vi "Synchronize Control Panel.vi"(8 "error in (no error)":errorcluster, 11 "Device in":refnum<class "Cryo-Con-22C.lvclass">) -> (0 "error out":errorcluster, 3 "Device out":refnum<class "Cryo-Con-22C.lvclass">)   [LabVIEW 2015, in "Cryo-Con-22C.lvclass"]
uses:
  Cryo-Con-22C.lvclass
  Cryo-Con Front Panel Data.ctl
  Cryo-con Heater Ranges.ctl
  Cry-Con Loop Type.ctl
  Instrument/Read VISA Resource.vi
  Instrument/Write VISA Resource.vi
  OO Devices/Device/Device.lvclass
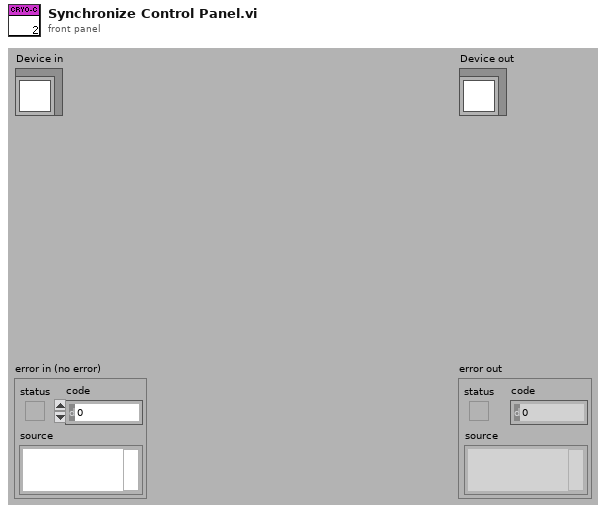
[diagram p1: front panel]
types:
  T1 = typedef "Cryo-Con Front Panel Data.ctl" = cluster{"Channels to measure":string[], "Record heater":bool, "Set point":dbl, "Heater Range":T2, "Control":bool, "Loop type":T3, "Ramp rate,\n K/min":dbl, "Control Channel":string, "P":dbl, "I":dbl, "D":dbl, "Manual %":u16}
  T2 = typedef "Cryo-con Heater Ranges.ctl" = enum16{"25W", "2.5W", "0.25W"}
  T3 = typedef "Cry-Con Loop Type.ctl" = enum16{"Off", "PID", "Manual", "PID Table", "PID Ramp", "PID Table Ramp"}
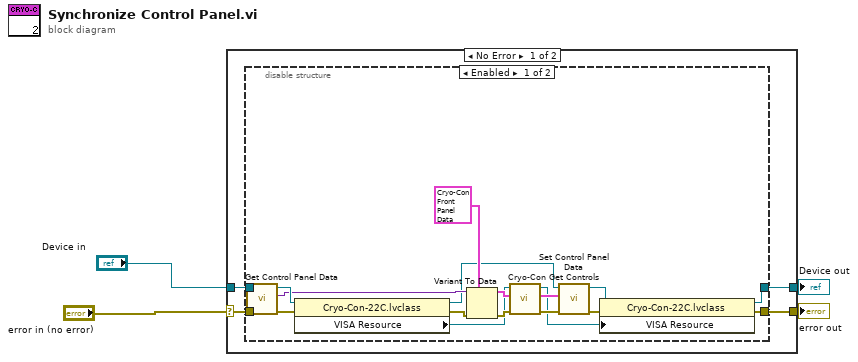
[diagram p0: block diagram]
diagram:
  n1 = case shown="No Error" "error in (no error)" {
    selector: "error in (no error)" -> [w7 w30]
    tunnel: [w6 w30] -> w3
    tunnel: [w5 w29] -> w1
    tunnel: "Device in" -> [w8 w29]
    frame No Error {
      n2 = disable-structure shown="Enabled" {
        disable-tunnel: w8 -> [w26 w27]
        disable-tunnel: w7 -> [w23 w28]
        disable-tunnel: [w15 w28] -> w6
        disable-tunnel: [w11 w27] -> w5
        frame Enabled {
          n3 = call-dynamic "Get Control Panel Data.vi"("error in (no error)"=w23, "Device in"=w26) -> ("error out"=w17:errorcluster, "Data"=w20:variant, "Device out"=w25:refnum<class "Cryo-Con-22C.lvclass">)  [unwired: 7 in]
          n4 = property class="Cryo-Con-22C.lvclass"(reference=w25, error in=w17) -> (reference out=w14:refnum<class "Cryo-Con-22C.lvclass">, error out=w16:errorcluster, "VISA Resource"=w9:refnum<visa-resource-name>)
          n5 = Variant To Data(error in=w16, type=T1 {"Channels to measure"=["A"], "Record heater"=FALSE, "Set point"=0.0, "Heater Range"=enum."25W", "Control"=FALSE, "Loop type"=enum."Off", "Ramp rate,\n K/min"=1.0, "Control Channel"="A", "P"=0.0, "I"=0.0, "D"=0.0, "Manual %"=0} ("Front Panel Data"), Variant=w20) -> (data=w21:T1, error out=w22:errorcluster)
          n6 = call "Cryo-Con Get Controls.vi"("error in (no error)"=w22, "Control Panel Data"=w21, "VISA resource name"=w9) -> ("error out"=w19:errorcluster, "Control Panel Data Out"=w18:T1, "VISA Resource Name Out"=w10:refnum<visa-resource-name>)  [unwired: 6 in]
          n7 = call "Set Control Panel Data.vi"("error in (no error)"=w19, "Data"=w18, "Device in"=w14) -> ("error out"=w12:errorcluster, "Device out"=w13:refnum<class "Cryo-Con-22C.lvclass">)  [unwired: 7 in]
          n8 = property class="Cryo-Con-22C.lvclass"(reference=w13, error in=w12, "VISA Resource"=w10) -> (reference out=w11:refnum<class "Cryo-Con-22C.lvclass">, error out=w15:errorcluster)
        }
        frame Disabled {
        }
      }
    }
    frame Error {
    }
  }
  "error out" <- w3
  "Device out" <- w1
